vi "niRFUtil MT UTIL IQ Impairments Axis Shear.vi"(0 "Waveform In":T1={"x0"=0.0, "dx"=1.0, "y"=[]} caption="input complex waveform" {"y" format="%.2f"; "dx" format="%^.2e"; "x0" format="%^.2e"}, 2 "IQ Gain Imbalance, dB":dbl format="%.2f", 3 "Quadrature Skew, degrees":dbl format="%.2f", 11 "error in (no error)":errorcluster) -> (4 "Waveform Out":T1 caption="output complex waveform" {"y" format="%.2f"; "dx" format="%^.2e"; "x0" format="%^.2e"}, 15 "error out":errorcluster)   [LabVIEW 2015, in "niRFUtil.lvlib"]
doc: "Performs the Gain Imbalance operation for IQ Impairment of an Input Data Waveform."
uses:
  niRFUtil.lvlib
  Includes/niRFUtil INC Complex Waveform.ctl
  Includes/niRFUtil INC Complex Array.ctl
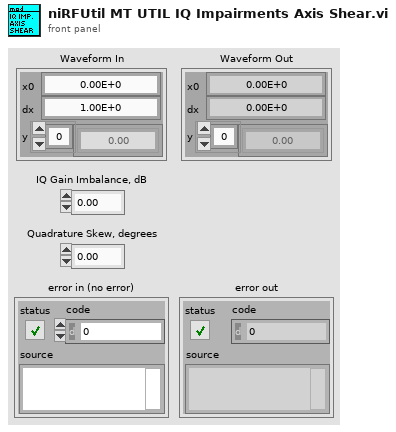
[diagram p1: front panel]
types:
  T1 = typedef "niRFUtil.lvlib/niRFUtil INC Complex Waveform.ctl" = cluster{"x0":dbl, "dx":dbl, "y":T2}
  T2 = typedef "niRFUtil.lvlib/niRFUtil INC Complex Array.ctl" = csg[]
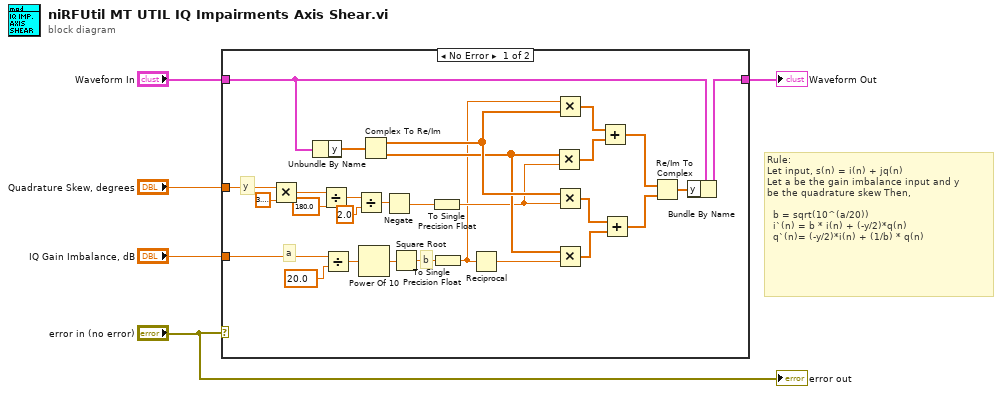
[diagram p0: block diagram]
diagram:
  # "Rule:\nLet input, s(n) = i(n) + jq(n)\nLet a be the gain imbalance input and y \nbe the quadrature skew Then,\n\n  b = sqrt(10^(a/20))\n  i`(n) = b * i(n) + (-y/2)*q(n)\n  q`(n)= (-y/2)*i(n) + (1/b) * q(n)"
  n1 = case shown="No Error" "error in (no error)" {
    tunnel: "IQ Gain Imbalance, dB" -> [w29 _]
    tunnel: "Waveform In" -> [w31 w34]
    tunnel: [w30 w34] -> w2
    tunnel: "Quadrature Skew, degrees" -> [w22 _]
    frame No Error {
      # "y"
      # "a"
      # "b"
      n2 = Multiply(x=w22, y=3.141592653589793) -> (x*y=w21:dbl)
      n3 = Unbundle By Name(w31) -> ("y"=w28:T2)
      n4 = Divide(x=w21, y=180.0) -> (x/y=w18:dbl)
      n5 = Divide(x=w29, y=20.0) -> (x/y=w32:dbl)
      n6 = Divide(x=w18, y=2.0) -> (x/y=w16:dbl)
      n7 = Power Of 10(x=w32) -> (10^x=w15:dbl)
      n8 = Complex To Re/Im(x + iy=w28) -> (x=w13:sgl[], y=w10:sgl[])
      n9 = Negate(x=w16) -> (-x=w9:dbl)
      n10 = Square Root(x=w15) -> (sqrt(x)=w14:dbl)
      n11 = To Single Precision Float(number=w9) -> (single precision float=w8:sgl)
      n12 = To Single Precision Float(number=w14) -> (single precision float=w6:sgl)
      n13 = Reciprocal(x=w6) -> (1/x=w7:sgl)
      n14 = Multiply(x=w10, y=w8) -> (x*y=w12:sgl[])
      n15 = Multiply(x=w6, y=w13) -> (x*y=w25:sgl[])
      n16 = Multiply(x=w13, y=w8) -> (x*y=w11:sgl[])
      n17 = Multiply(x=w10, y=w7) -> (x*y=w26:sgl[])
      n18 = Add(x=w25, y=w12) -> (x+y=w24:sgl[])
      n19 = Add(x=w11, y=w26) -> (x+y=w23:sgl[])
      n20 = Re/Im To Complex(1:w23, 2:w24) -> (0:w27:csg[])
      n21 = Bundle By Name(cluster=w31, "y"=w27) -> (w30:T1)
    }
    frame Error {
    }
  }
  "Waveform Out" <- w2
  "error out" <- "error in (no error)"
